vi "Regler Pumpe nur Drehzahl.vi"(8 "Fehler":errorcluster caption="Fehler (Eingang)") -> (0 "Fehler (Ausgang)":errorcluster)   [LabVIEW 2020, in "Regler.lvlib" / "Druckregler.lvlib"]
uses:
  Druckregler.lvlib
  Konfig-Dateien/FGV Betriebsdaten Aktionen.ctl
  Verwaltung/FGV OUT Aktionen.ctl
  Verwaltung/Verwaltung - cRIO.lvlib
  Konfig-Dateien/Konfig-Dateien.lvlib
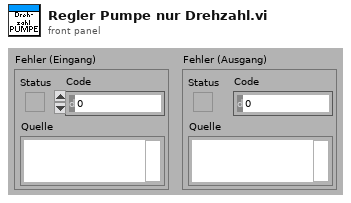
[diagram p1: front panel]
types:
  T1 = typedef "Verwaltung - cRIO.lvlib/FGV OUT Aktionen.ctl" = enum16{"lesen", "ANA OUT", "DO 0-31", "DO 32-47"}
  T2 = typedef "Konfig-Dateien.lvlib/FGV Betriebsdaten Aktionen.ctl" = enum16{"lesen", "Anlagengrenzw.", "PID Param.", "Sonstige", "Sensor Para."}
  T3 = typedef "Erweiterte Konfig.lvlib/Sonstige Parameter.ctl" = cluster{"Lüfter langsam":sgl, "Lüfter schnell":sgl, "FT-IR Kühlung Soll":sgl, "FT-IR Kühlung Max":sgl, "Überwachung":T4, "Befüllung aktiv":T5, "Stickstoff Befüllzeit":sgl, "Befüllintervall":sgl, "Kalibrierwert FT-IR":sgl, "Offset Ausgang":sgl, "Offset FT-IR":sgl, "Offset Druck FT-IR":sgl, "Dichtheitstest Zeit":sgl, "Dichtheitstest Abfall":sgl, "Dichtheitstest Umfang":T6, "Offset Umgebung":sgl, "Max Taupunkt":sgl, "Pumpendrehzahl":sgl, "ext. Befüllung":T5, "Ext. Stickstoff Befüllzeit":sgl}
  T4 = typedef "Auswahlfeld.ctl" = u16
  T5 = typedef "LogKonfig.lvlib/Auswahlfeld aktiviert-deaktiviert.ctl" = u16
  T6 = typedef "Erweiterte Konfig.lvlib/Dichtheitstest Umfang.ctl" = u16
  T7 = typedef "Verwaltung - cRIO.lvlib/Digital Ausgaenge 32-63.ctl" = cluster{"O32: Messgaspumpe EIN":bool, "O33: (Umgebungsluftpumpe)":bool, "O34: (Kondensatpumpe GK)":bool, "O35: Klima/Lüfter EIN":bool, "O36: Versorgung Heizungen":bool, "O37: Versorgung Heizungen":bool, "O38: (Gaskühler EIN (Freigabe))":bool, "O39: Störung FAS LP":bool, "O40: (Heizung Filterblock)":bool, "O41: Heizung HL zu FT-IR":bool, "O42: Heizung HL Extern SP1":bool, "O43: Heizung HL Extern SP2":bool, "O44: Heizung Reserve":bool, "O45: Heizung Reserve":bool, "O46: Statusbeleuchtung grün":bool, "O47: Statusbeleuchtung rot":bool}
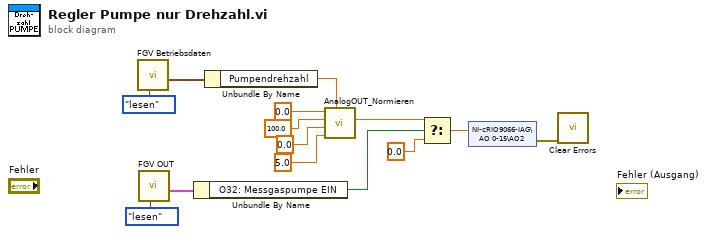
[diagram p0: block diagram]
diagram:
  n1 = call "FGV Betriebsdaten.vi"("Aktionen"=FGV_Betriebsdaten_Aktionen."lesen") -> ("Sonstige"=w8:T3)  [unwired: 7 in, 3 out]
  n2 = call "FGV OUT.vi"("Aktion"=FGV_OUT_Aktionen."lesen") -> ("DO 32-63"=w9:T7)  [unwired: 7 in, 3 out]
  n3 = Unbundle By Name(w9) -> ("O32: Messgaspumpe EIN"=w3:bool)
  n4 = Unbundle By Name(w8) -> ("Pumpendrehzahl"=w6:sgl)
  n5 = call "AnalogOUT_Normieren.vi"("Analogwert"=w6, "Obergrenze"=sgl 5.0, "Untergrenze"=sgl 0.0, "Max Analogwert"=sgl 100.0, "Min Analogwert"=sgl 0.0) -> ("Normierter Wert"=w5:sgl)  [unwired: 6 in]
  n6 = Select(t=w5, s=w3, f=sgl 0.0) -> (s? t:f=w2:sgl)
  n7 = shared-variable "NI-cRIO9066-IAG\\AO 0-15\\AO2"(w2) -> (error out=w1:errorcluster)  [unwired: 1 in]
  n8 = call <vilib>:"Clear Errors.vi"("error in (no error)"=w1) -> ()  [unwired: 5 in, 2 out]
